vi "globalSetUp.vi"(8 "error in":errorcluster, 11 "Single Board Loopback in":refnum<class "Single Board 1Ch Loopback.lvclass">) -> (0 "error out":errorcluster, 3 "Single Board Loopback out":refnum<class "Single Board 1Ch Loopback.lvclass">)   [LabVIEW 2020, in "Single Board 1Ch Loopback.lvclass"]
uses:
  Single Board 1Ch Loopback.lvclass
  Single Board 1Ch Loopback.lvclass/Single Board 1Ch Loopback.ctl
  niveristand-custom-device-testing-tools/VeriStandTestUtilities/VeriStandTestUtilities.lvlib
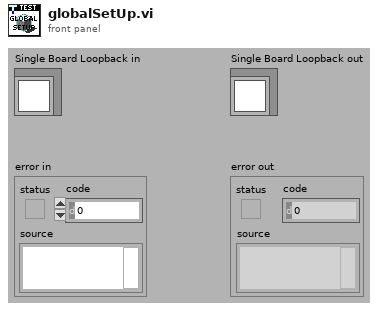
[diagram p1: front panel]
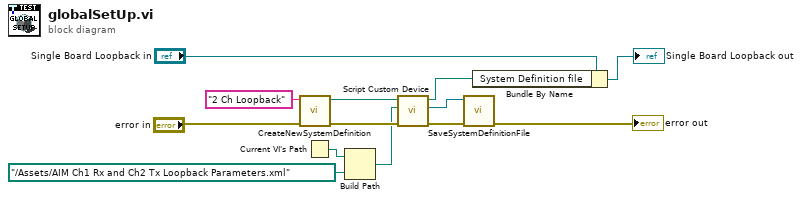
[diagram p0: block diagram]
diagram:
  n1 = call "CreateNewSystemDefinition.vi"("error in"="error in", "System Definition Name"="2 Ch Loopback" ("Channel")) -> ("error out"=w9:errorcluster, "System Definition Path"=w8:path)  [unwired: 8 in]
  n2 = Current VI's Path() -> (path=w13:path)
  n3 = Build Path(base path=w13, name or relative path=path "../Assets/AIM Ch1 Rx and Ch2 Tx Loopback Parameters.xml") -> (appended path=w5:path)
  n4 = call "Script Custom Device.vi"("error in"=w9, "Parameter File Path"=w5, "System Definition File Path In"=w8) -> ("error out"=w12:errorcluster, "System Definition Reference"=w6:refnum<k24>, "System Definition File Path Out"=w2:path)  [unwired: 5 in, 1 out]
  n5 = call "SaveSystemDefinitionFile.vi"("error in (no error)"=w12, "System Definition Reference in"=w6) -> ("error out"=→"error out":errorcluster)  [unwired: 8 in, 1 out]
  n6 = Bundle By Name(cluster="Single Board Loopback in", "System Definition file"=w2) -> (→"Single Board Loopback out":refnum<class "Single Board 1Ch Loopback.lvclass">)
